vi "PDE Thermal Distribution_RHS.vi"(2 "data":variant, 3 "y":dbl, 4 "x":dbl, 5 "t":dbl) -> (0 "error out":errorcluster, 1 "F(t, x, y)":dbl)   [LabVIEW 2023]
doc: "This VI implements the right side of the equation."
panel:
  # "This is an example of a VI that the PDE solver can call by reference. All VIs called by the PDE solver must have the same connector pane."
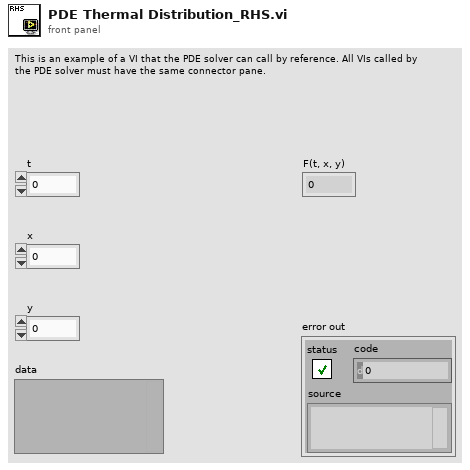
[diagram p1: front panel]
types:
  T1 = cluster{"Amp":dbl, "Center X":dbl, "Center Y":dbl, "Std X":dbl, "Std Y":dbl}
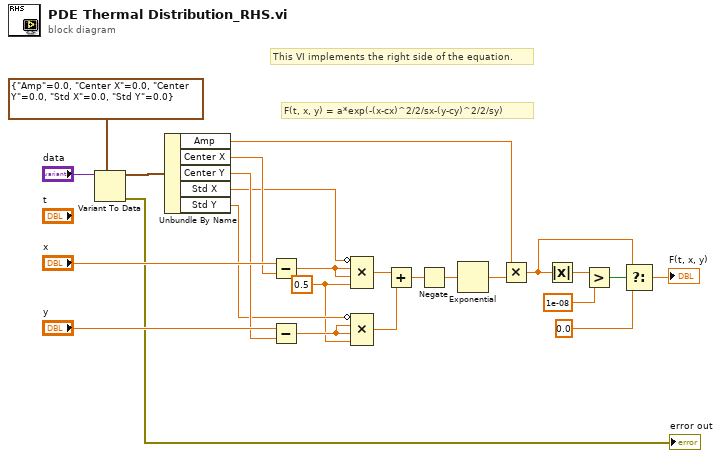
[diagram p0: block diagram]
diagram:
  w14 = 0.5 ("value")
  # "This VI implements the right side of the equation."
  # "F(t, x, y) = a*exp(-(x-cx)^2/2/sx-(y-cy)^2/2/sy)"
  n1 = Variant To Data(type=T1 {"Amp"=0.0, "Center X"=0.0, "Center Y"=0.0, "Std X"=0.0, "Std Y"=0.0}, Variant="data") -> (data=w23:T1, error out=→"error out":errorcluster)  [unwired: 1 in]
  n2 = Unbundle By Name(w23) -> ("Amp"=w8:dbl, "Center X"=w21:dbl, "Center Y"=w19:dbl, "Std X"=w17:dbl, "Std Y"=w16:dbl)
  n3 = Subtract(x="x", y=w21) -> (x-y=w18:dbl)
  n4 = Subtract(x="y", y=w19) -> (x-y=w15:dbl)
  n5 = Compound Arithmetic op=MULTIPLY(invert w17, w18, w18, w14) -> (w13:dbl)
  n6 = Compound Arithmetic op=MULTIPLY(invert w16, w15, w15, w14) -> (w12:dbl)
  n7 = Add(x=w13, y=w12) -> (x+y=w11:dbl)
  n8 = Negate(x=w11) -> (-x=w10:dbl)
  n9 = Exponential(1:w10) -> (0:w9:dbl)
  n10 = Multiply(x=w8, y=w9) -> (x*y=w4:dbl)
  n11 = Absolute Value(x=w4) -> (abs(x)=w7:dbl)
  n12 = Greater?(x=w7, y=1e-08) -> (0:w5:bool)
  n13 = Select(t=w4, s=w5, f=0.0) -> (s? t:f=→"F(t, x, y)":dbl)
